vi "begin.vi"(8 "error in (no error)":errorcluster, 9 "blinkingEnabledIsTrue (F)":bool, 10 "alarmTreeRefnum":refnum<vi>, 11 "AlarmsTreeDisplayTC in":refnum<class "AlarmsTreeDisplayTC.lvclass">) -> (0 "error out":errorcluster, 3 "AlarmsTreeDisplayTC out":refnum<class "AlarmsTreeDisplayTC.lvclass">)   [LabVIEW 2012, in "AlarmsTreeDisplayTC.lvclass"]
doc: "Begins execution of the alarms tree display; initializes object and calls the start method on the parent."
uses:
  AlarmsTreeDisplayTC.lvclass
  C/Program Files (x86)/National Instruments/LabVIEW 2012/user.lib/Common/AlarmsTreeDisplay/AlarmsTreeDisplay/AlarmsTreeDisplay.lvclass
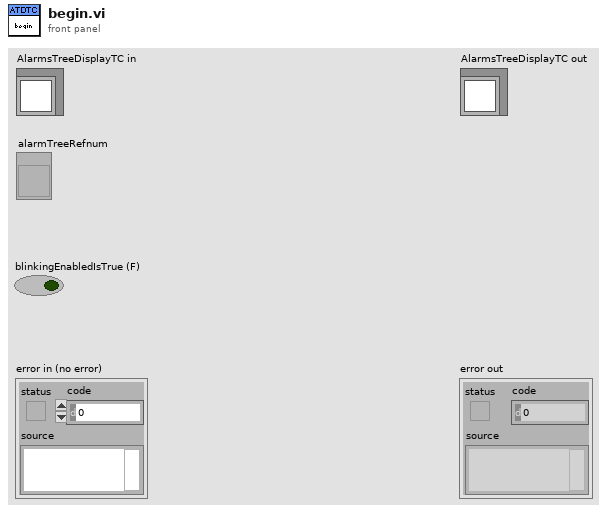
[diagram p1: front panel]
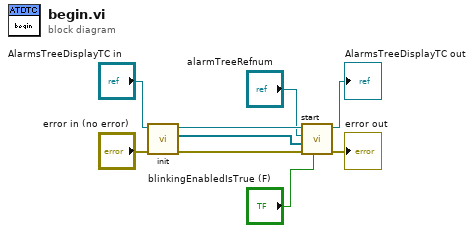
[diagram p0: block diagram]
diagram:
  n1 = call "init.vi"("error in (no error)"="error in (no error)", "AlarmsTreeDisplayTC in"="AlarmsTreeDisplayTC in") -> ("error out"=w5:errorcluster, "shared variables"=w6:refnum<k21>[], "AlarmsTreeDisplayTC out"=w8:refnum<class "AlarmsTreeDisplayTC.lvclass">)  [unwired: 7 in]
  n2 = call "start.vi"("blinkingEnabledIsTrue (F)"="blinkingEnabledIsTrue (F)", "error in (no error)"=w5, "shared variables"=w6, "alarmTreeRefnum"="alarmTreeRefnum", "AlarmsTreeDisplay in"=w8) -> ("error out"=→"error out":errorcluster, "AlarmsTreeDisplay out"=→"AlarmsTreeDisplayTC out":refnum<class "AlarmsTreeDisplayTC.lvclass">)  [unwired: 5 in]
